vi "MSG Read Controller Input.vi"(8 "error in":errorcluster) -> (0 "error out":errorcluster)   [LabVIEW 2020, in "Hardware.lvlib"]
uses:
  Hardware.lvlib
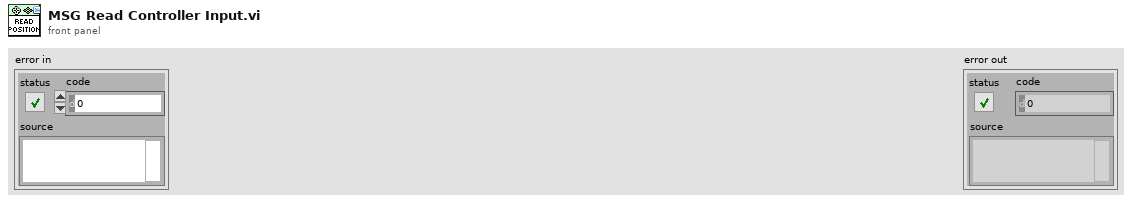
[diagram p1: front panel]
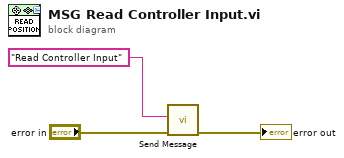
[diagram p0: block diagram]
diagram:
  n1 = call "Send Message.vi"("error in"="error in", "Command"="Read Controller Input") -> ("error out"=→"error out":errorcluster)  [unwired: 9 in]
